vi "GetText.vi"(8 "error in":errorcluster, 11 "node in":refnum<class "RunTimeMenuItem.lvclass">) -> (0 "error out":errorcluster, 1 "additional text":string, 2 "text":string, 3 "node out":refnum<class "RunTimeMenuItem.lvclass">, 4 "glyph":string)   [LabVIEW 2015, in "RunTimeMenuItem.lvclass"]
doc: "Returns the text representation of the node used for the tree control."
uses:
  RunTimeMenuItem.lvclass
  RunTimeMenuItem.lvclass/RunTimeMenuItem.ctl
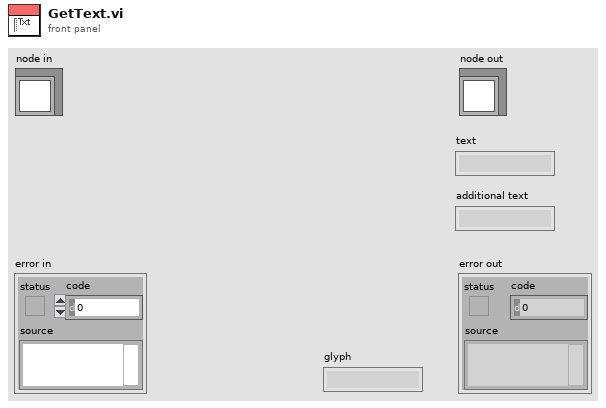
[diagram p1: front panel]
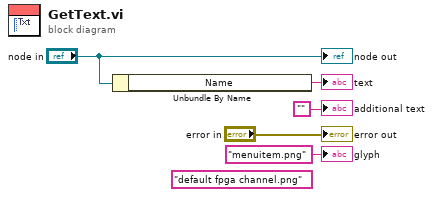
[diagram p0: block diagram]
diagram:
  (unwired) "default fpga channel.png" ("glyph")
  n1 = Unbundle By Name("node in") -> ("Name"=→"text":string)
  "error out" <- "error in"
  "node out" <- "node in"
  "additional text" <- ""
  "glyph" <- "menuitem.png" ("glyph")
